vi "ActiveX.vi"() -> ()   [LabVIEW 2014]
panel:
  in  "URL":string
  in  "WebBrowser":refnum<k7>(container)
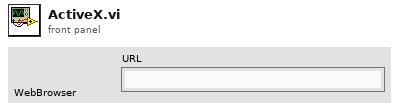
[diagram p1: front panel]
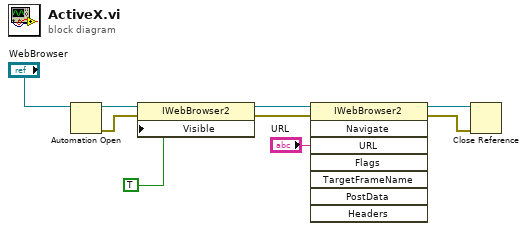
[diagram p0: block diagram]
diagram:
  n1 = Automation Open(Automation Refnum="WebBrowser") -> (Automation Refnum=w9:refnum<k7>, error out=w6:errorcluster)  [unwired: 3 in]
  n2 = property on="프로퍼티 노드" class="IWebBrowser2"(reference=w9, error in=w6, "Visible"=TRUE) -> (reference out=w8:refnum<k7>, error out=w5:errorcluster)
  n3 = invoke on="인보크 노드" class="IWebBrowser2" method="Navigate"(reference=w8, error in=w5, "URL"="URL") -> (reference out=w7:refnum<k7>, error out=w4:errorcluster)  [unwired: 5 in, 6 out]
  n4 = Close Reference(reference=w7, error in (no error)=w4) -> ()  [unwired: 1 out]
